vi "get_graph_reference.vi"(8 "error in (no error)":errorcluster, 9 "raw channel index":i32, 11 "DisplayDL090216 in":refnum<class "DisplayDL090216.lvclass">) -> (0 "error out":errorcluster, 1 "histogram reference out":refnum<vi>, 3 "DisplayDL090216 out":refnum<class "DisplayDL090216.lvclass">)   [LabVIEW 2010, in "DisplayDL090216.lvclass"]
uses:
  DisplayDL090216.lvclass
  DisplayDL090216.lvclass/DisplayDL090216.ctl
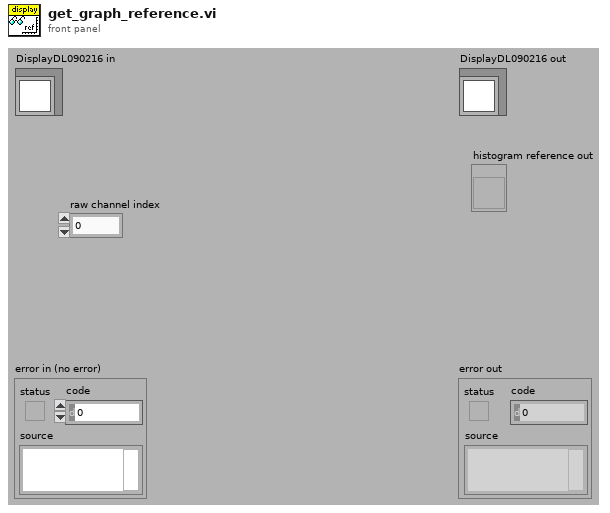
[diagram p1: front panel]
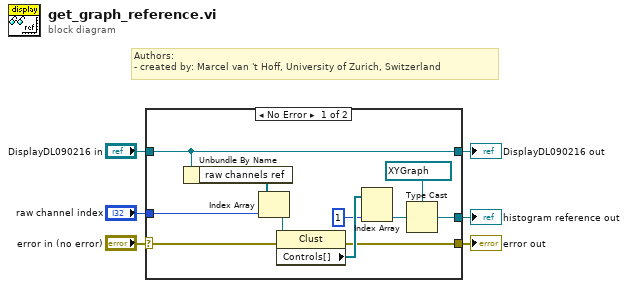
[diagram p0: block diagram]
diagram:
  # "Authors: \n- created by: Marcel van 't Hoff, University of Zurich, Switzerland"
  n1 = case shown="No Error" "error in (no error)" {
    selector: "error in (no error)" -> [w13 w19]
    tunnel: [w7 w19] -> w3
    tunnel: [w14 w18] -> w2
    tunnel: "DisplayDL090216 in" -> [w14 w18]
    tunnel: "raw channel index" -> [w12 _]
    tunnel: [w8 _] -> w1
    frame No Error {
      n2 = Unbundle By Name(w14) -> ("raw channels ref"=w16:refnum<vi>[])
      n3 = Index Array(array=w16, index=w12) -> (element=w17:refnum<vi>)
      n4 = property class="Clust"(reference=w17, error in=w13) -> (error out=w7:errorcluster, "Controls[]"=w15:refnum<vi>[])  [unwired: 1 out]
      n5 = Index Array(array=w15, index #2=1 ("index")) -> (element #2=w11:refnum<vi>)  [unwired: 1 in, 1 out]
      n6 = Type Cast(type=refnum<vi> refnum ("histogram out"), x=w11) -> (*(type *) &x=w8:refnum<vi>)
    }
    frame Error {
    }
  }
  "error out" <- w3
  "DisplayDL090216 out" <- w2
  "histogram reference out" <- w1
